vi "test-AttrMap-NotExistButTrytoFind.vi"(8 "error in (no error)":errorcluster, 11 "TestCase in":refnum<class "MyTestCase.lvclass">) -> (0 "error out":errorcluster, 3 "TestCase out":refnum<class "MyTestCase.lvclass">)   [LabVIEW 2019, in "MyTestCase.lvclass"]
uses:
  MyTestCase.lvclass
  c69e2828-ad39-4405-adde-a0dbf068bb39.vi
  c69e2828-ad39-4405-adde-a0dbf068bb39.vi/facf7ccb-bfaf-4d49-89ba-510e3f52c677.vi
  src/API/AttrMap/RawAttrMap.vi
  src/_Support/__AttrMap-GetValue2.vi
  src/API/VAttributes/VAttrbutesToData.vi
  src/_Support/__AttrMap-SetValue2.vi
  src/API/AttrMap/AttrMap-Merge.vi
  <vilib>/addons/_JKI Toolkits/VI Tester/TestCase.llb/TestCase.lvclass
  C:/Program Files (x86)/National Instruments/LabVIEW 2019/vi.lib/addons/_JKI Toolkits/VI Tester/TestCase.llb/TestCase.lvclass
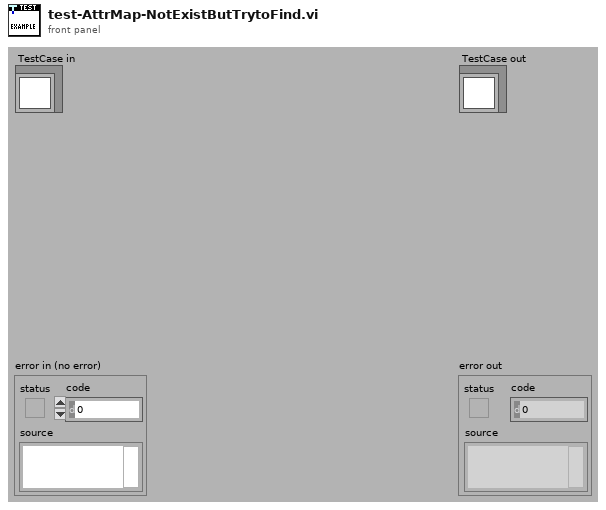
[diagram p1: front panel]
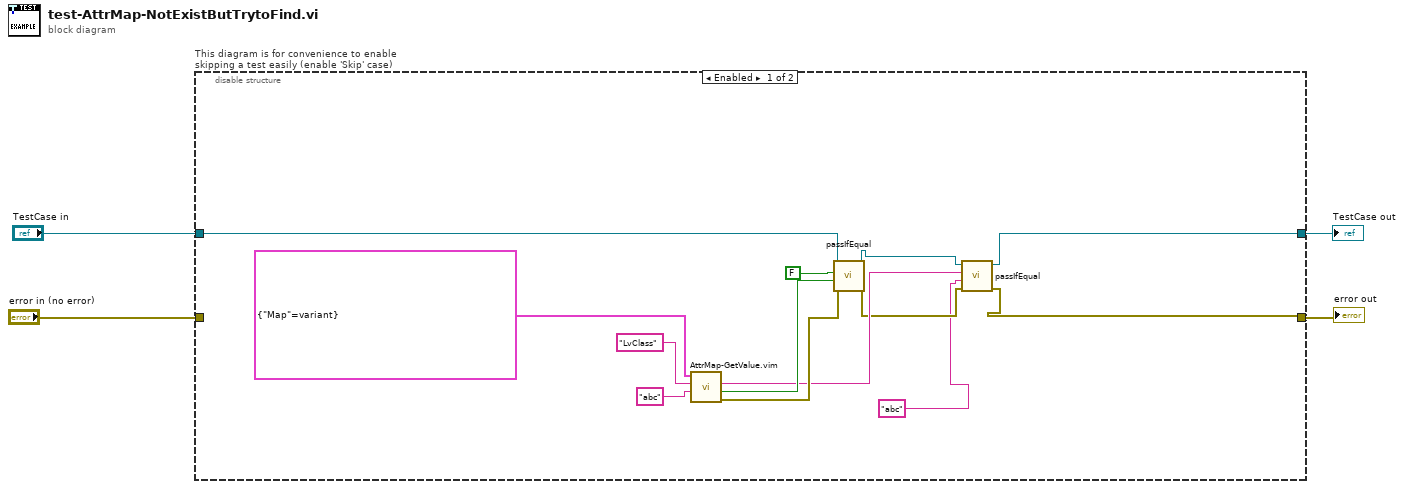
[diagram p0: block diagram]
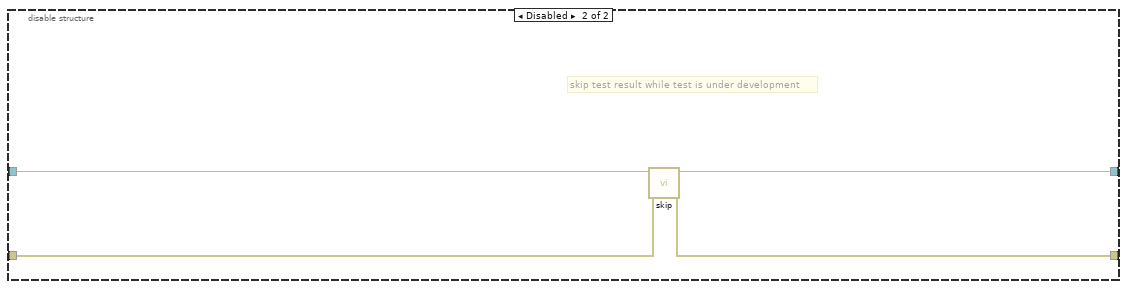
[diagram p2: hidden frame]
diagram:
  n1 = disable-structure "This diagram is for convenience to enable skipping a test easily (enable 'Skip' case)" shown="Enabled" {
    disable-tunnel: "TestCase in" -> [w17 w21]
    disable-tunnel: [w8 w19] -> w1
    disable-tunnel: [w6 w20] -> w3
    disable-tunnel: "error in (no error)" -> [_ w18]
    frame Enabled {
      n2 = call "AttrMap-GetValue.vim"("DefaultValue"="abc" ("Key(String/Enum)"), "Key(String/Enum)"="LvClass", "AttrMap in"=cluster{"Map":variant} {"Map"=variant(variant[] [variant("name"=variant(string "Name"))], "name"=variant(string "HAL_ABC_LV2_MODIFY_IN_JSON"))} ("HALAttrMap")) -> ("error out"=w15:errorcluster, "found"=w14:bool, "Value"=w10:string)  [unwired: 4 in, 2 out]
      n3 = call-dynamic "passIfEqual.vi"("error in (no error)"=w15, "y"=w14, "x"=FALSE ("found"), "TestCase in"=w17) -> ("error out"=w7:errorcluster, "TestCase out"=w9:refnum<class "MyTestCase.lvclass">)  [unwired: 6 in]
      n4 = call-dynamic "passIfEqual.vi"("error in (no error)"=w7, "y"="abc" ("Key(String/Enum)"), "x"=w10, "TestCase in"=w9) -> ("error out"=w6:errorcluster, "TestCase out"=w8:refnum<class "MyTestCase.lvclass">)  [unwired: 6 in]
    }
    frame Disabled {
      # "skip test result while test is under development"
      n5 = call <vilib>:"skip.vi"("error in (no error)"=w18, "TestCase in"=w21) -> ("error out"=w20:errorcluster, "TestCase out"=w19:refnum<class "MyTestCase.lvclass">)  [unwired: 8 in]
    }
  }
  "error out" <- w3
  "TestCase out" <- w1
